vi "getData.vi"(8 "error in (no error)":errorcluster, 11 "RampEvent in":refnum<class "RampEvent.lvclass">) -> (0 "error out":errorcluster, 1 "dataType":T1(ring), 2 "data":T2 {"times" format="%#_19g"}, 3 "RampEvent out":refnum<class "RampEvent.lvclass">)   [LabVIEW 2011, in "Tools.lvlib" / "Scripting.lvlib" / "RampEvent.lvclass"]
uses:
  RampEvent.lvclass
  DatabaseHelpers/Database Objects/Channel/Channel.lvclass
  RampEvent.lvclass/RampEvent.ctl
  ScriptEvent.lvclass
panel:
  out "samples":i32
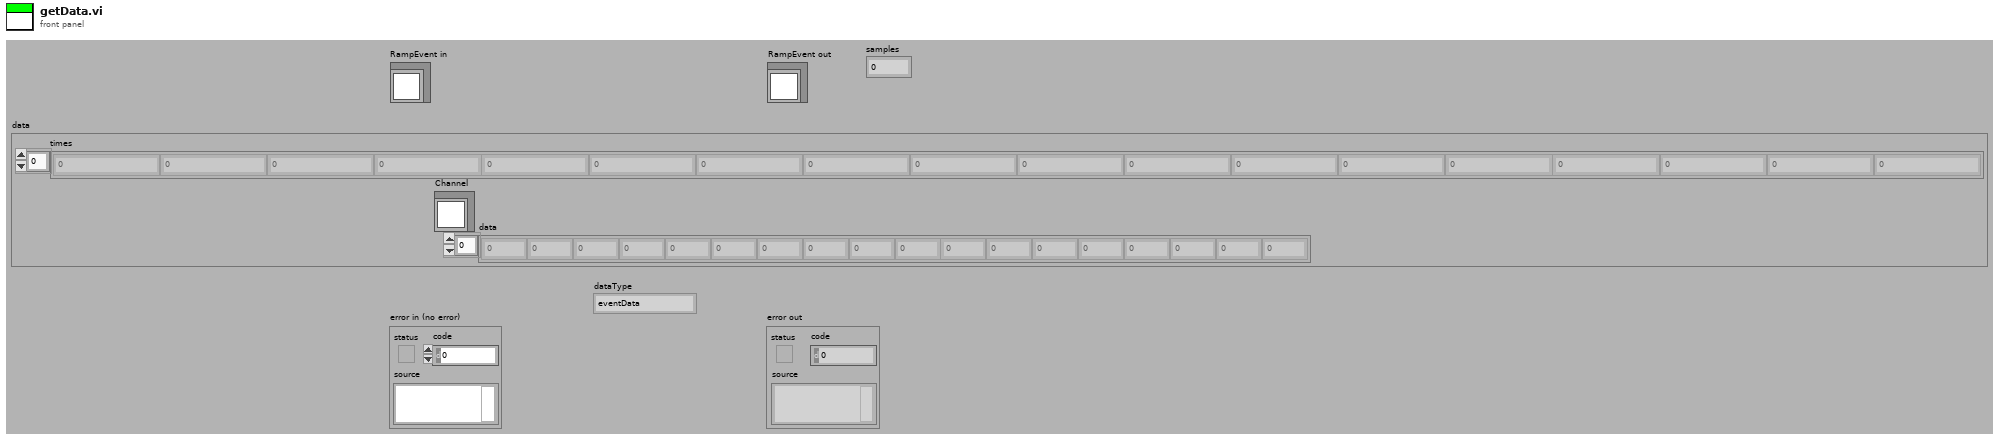
[diagram p1: front panel]
types:
  T1 = enum16{"eventData", "singleToneData", "fileData"}
  T2 = cluster{"times":dbl[], "Channel":refnum<class "Channel.lvclass">, "data":dbl[]}
  T3 = cluster{dbl[], "Channel.lvclass":refnum<class "Channel.lvclass">, dbl[]}
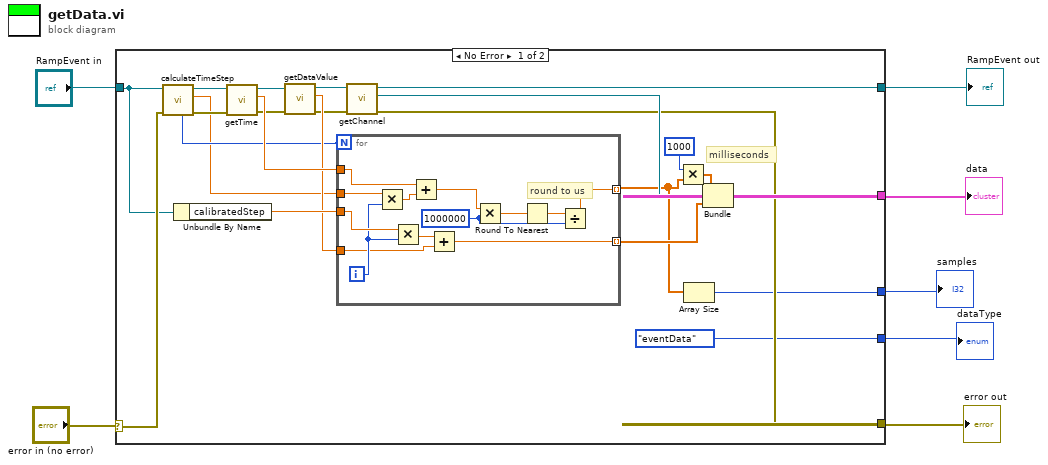
[diagram p0: block diagram]
diagram:
  n1 = case shown="No Error" "error in (no error)" {
    selector: "error in (no error)" -> [w30 w44]
    tunnel: [w18 w45] -> w7
    tunnel: "RampEvent in" -> [w29 w45]
    tunnel: [w16 w44] -> w4
    tunnel: [w19 _] -> w3
    tunnel: [T1."eventData" ("dataType") _] -> w2
    tunnel: [w9 _] -> w1
    frame No Error {
      # "milliseconds"
      n2 = call "calculateTimeStep.vi"("error in (no error)"=w30, "RampEvent in"=w29) -> ("error out"=w27:errorcluster, "timeStep"=w8:dbl, "RampEvent out"=w28:refnum<class "RampEvent.lvclass">, "number of Steps"=w12:i32)  [unwired: 5 in, 1 out]
      n3 = Unbundle By Name(w29) -> ("calibratedStep"=w25:dbl)
      n4 = call "getTime.vi"("error in (no error)"=w27, "ScriptEvent.lvclass in"=w28) -> ("error out"=w23:errorcluster, "time"=w26:dbl, "ScriptEvent.lvclass out"=w24:refnum<class "RampEvent.lvclass">)  [unwired: 7 in]
      n5 = call "getDataValue.vi"("error in (no error)"=w23, "ScriptEvent.lvclass in"=w24) -> ("error out"=w21:errorcluster, "dataValue"=w22:dbl, "ScriptEvent.lvclass out"=w20:refnum<class "RampEvent.lvclass">)  [unwired: 7 in]
      n6 = for {
        N: w12 -> [_]
        tunnel: w26 -> [w42]
        tunnel: w8 -> [w43]
        tunnel: w25 -> [w40]
        tunnel: w22 -> [w37]
        tunnel: [w31] -> w10 mode=indexing
        tunnel: [w36] -> w11 mode=indexing
        i -> [w39]
        w33 = 1000000
        # "round to us"
        n7 = Multiply(x=w43, y=w39) -> (x*y=w41:dbl)
        n8 = Multiply(x=w40, y=w39) -> (x*y=w38:dbl)
        n9 = Add(x=w42, y=w41) -> (x+y=w32:dbl)
        n10 = Add(x=w38, y=w37) -> (x+y=w36:dbl)
        n11 = Multiply(x=w32, y=w33) -> (x*y=w35:dbl)
        n12 = Round To Nearest(number=w35) -> (nearest integer value=w34:dbl)
        n13 = Divide(x=w34, y=w33) -> (x/y=w31:dbl)
      }
      n14 = call-dynamic "getChannel.vi"("error in (no error)"=w21, "ScriptEvent.lvclass in"=w20) -> ("error out"=w16:errorcluster, "Channel.lvclass"=w17:refnum<class "Channel.lvclass">, "ScriptEvent.lvclass out"=w18:refnum<class "RampEvent.lvclass">)  [unwired: 7 in]
      n15 = Multiply(x=1000, y=w10) -> (x*y=w15:dbl[])
      n16 = Array Size(array=w10) -> (size(s)=w9:i32)
      n17 = Bundle(w15, "Channel.lvclass"=w17, w11) -> (w19:T3)  [unwired: 1 in]
    }
    frame Error {
    }
  }
  "error out" <- w4
  "RampEvent out" <- w7
  "data" <- w3
  "dataType" <- w2
  "samples" <- w1
